vi "write_attributes.vi"(8 "error in (no error)":errorcluster, 10 "attributes":T1, 11 "LocallyLinearEmbedding in":refnum<class "LocallyLinearEmbedding.lvclass">) -> (0 "error out":errorcluster, 3 "LocallyLinearEmbedding out":refnum<class "LocallyLinearEmbedding.lvclass">)   [LabVIEW 2020, in "LocallyLinearEmbedding.lvclass"]
uses:
  LocallyLinearEmbedding.lvclass
  Controls/locally_linear_embedding_attributes.ctl
  LocallyLinearEmbedding.lvclass/LocallyLinearEmbedding.ctl
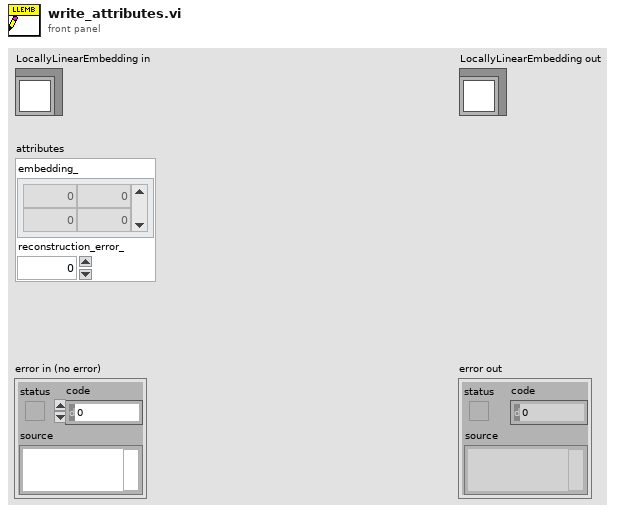
[diagram p1: front panel]
types:
  T1 = typedef "locally_linear_embedding_attributes.ctl" = cluster{"embedding_":dbl[][], "reconstruction_error_":dbl}
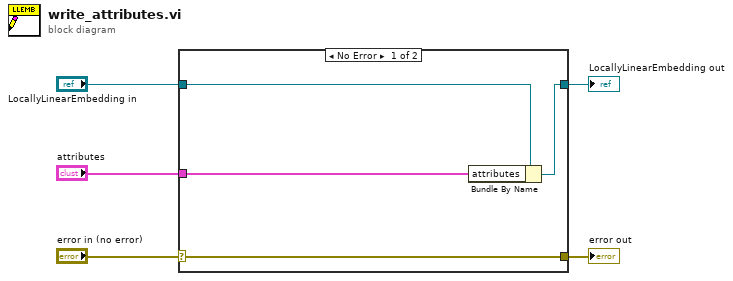
[diagram p0: block diagram]
diagram:
  n1 = case shown="No Error" "error in (no error)" {
    selector: "error in (no error)" -> [w9 w10]
    tunnel: [w9 w10] -> w4
    tunnel: [w7 w11] -> w2
    tunnel: "LocallyLinearEmbedding in" -> [w8 w11]
    tunnel: "attributes" -> [w6 _]
    frame No Error {
      n2 = Bundle By Name(cluster=w8, "attributes"=w6) -> (w7:refnum<class "LocallyLinearEmbedding.lvclass">)
    }
    frame Error {
    }
  }
  "error out" <- w4
  "LocallyLinearEmbedding out" <- w2
